vi "TAN to p2.vi"() -> ()   [LabVIEW 2009]
uses:
  <vilib>/printing/ReportDocExtensions.llb/Append Front Panel Image to Report (path).vi
  <vilib>/Utility/NIReport.llb/NI_report.lvclass
  <vilib>/Utility/NIReport.llb/NI_ReportGenerationCore.lvlib
panel:
  in  "Tab Control":enum32{"serving", "Receiving"}(tab)
  out "ALL":dbl[](graph)
  out "Left 2":dbl[](graph)
  out "Right 2":dbl[](graph)
  out "Serve 4":dbl[](graph)
  out "Serve 5":dbl[](graph)
  out "Serve 1":dbl[](graph)
  out "Serve 6":dbl[](graph)
  out "Serve 7":dbl[](graph)
  out "Serve 2":dbl[](graph)
  out "Serve 8":dbl[](graph)
  out "Serve 9":dbl[](graph)
  out "Serve 3":dbl[](graph)
  in  "S1":bool
  in  "TL":bool
  in  "BR":bool
  in  "BL":bool
  in  "BM":bool
  in  "CR":bool
  in  "CM":bool
  in  "CL":bool
  in  "TR":bool
  in  "TM":bool
  in  "1":bool
  in  "2":bool
  in  "3":bool
  in  "S 2":bool
  in  "Code":bool
  in  "stop":bool
  in  "save file to":path=path "C:/Users/Sports Tech/Desktop/kokum/Service VI/SAVED FILES/results.doc"
  in  "String":string
  in  "reset":bool
  in  "Boolean":bool
  in  "TM 3":bool
  in  "TR 3":bool
  in  "CL 3":bool
  in  "CM 3":bool
  in  "CR  3":bool
  in  "BM 3":bool
  in  "BL 3":bool
  in  "BR 3":bool
  in  "TL 3":bool
  in  "TM 2":bool
  in  "TR 2":bool
  in  "CL 2":bool
  in  "CM 2":bool
  in  "CR  2":bool
  in  "BM 2":bool
  in  "BL 2":bool
  in  "BR 2":bool
  in  "TL 2":bool
  out "All":dbl[](graph)
  out "Right":dbl[](graph)
  out "Left":dbl[](graph)
  out "Return 6":dbl[](graph)
  out "return to 9":dbl[](graph)
  out "return to 6":dbl[](graph)
  out "Return 7":dbl[](graph)
  out "return to 10":dbl[](graph)
  out "return to 7":dbl[](graph)
  out "Return 8":dbl[](graph)
  out "return to 11":dbl[](graph)
  out "return to 8":dbl[](graph)
  out "Return 0":dbl[](graph)
  out "return to 3":dbl[](graph)
  out "return to 0":dbl[](graph)
  out "Return 1":dbl[](graph)
  out "return to 4":dbl[](graph)
  out "return to 1":dbl[](graph)
  out "Return 2":dbl[](graph)
  out "return to 5":dbl[](graph)
  out "return to 2":dbl[](graph)
  out "return to 1 from right":dbl[][](array[numeric])
  out "return to 2 from right":dbl[][](array[numeric])
  out "return to 6 from right":dbl[][](array[numeric])
  out "return to 7 from right":dbl[][](array[numeric])
  out "return to 8 from right":dbl[][](array[numeric])
  out "return to 0 from right":dbl[][](array[numeric])
  out "return to 8 from left":dbl[][](array[numeric])
  out "return to 7 from left":dbl[][](array[numeric])
  out "return to 6 from left":dbl[][](array[numeric])
  out "return to 2 from left":dbl[][](array[numeric])
  out "return to 1 from left":dbl[][](array[numeric])
  out "return to 0 from left":dbl[][](array[numeric])
  out "All receives":dbl[][](array[numeric])
  out "receive from left":dbl[][](array[numeric])
  out "receive from right":dbl[][](array[numeric])
  out "serve3":dbl[][](array[numeric])
  out "serve2":dbl[][](array[numeric])
  out "serve1":dbl[][](array[numeric])
  out "serv1 from right":dbl[][](array[numeric])
  out "serv2 from right":dbl[][](array[numeric])
  out "serv3 from right":dbl[][](array[numeric])
  out "serv3 from left":dbl[][](array[numeric])
  out "serv2 from left":dbl[][](array[numeric])
  out "serv1 from left":dbl[][](array[numeric])
  out "all serves":dbl[][](array[numeric])
  out "service from right":dbl[][](array[numeric])
  out "serving from left":dbl[][](array[numeric])
  # "SWITCH"
  # "Receiving"
  # "Player position"
  # "Serving"
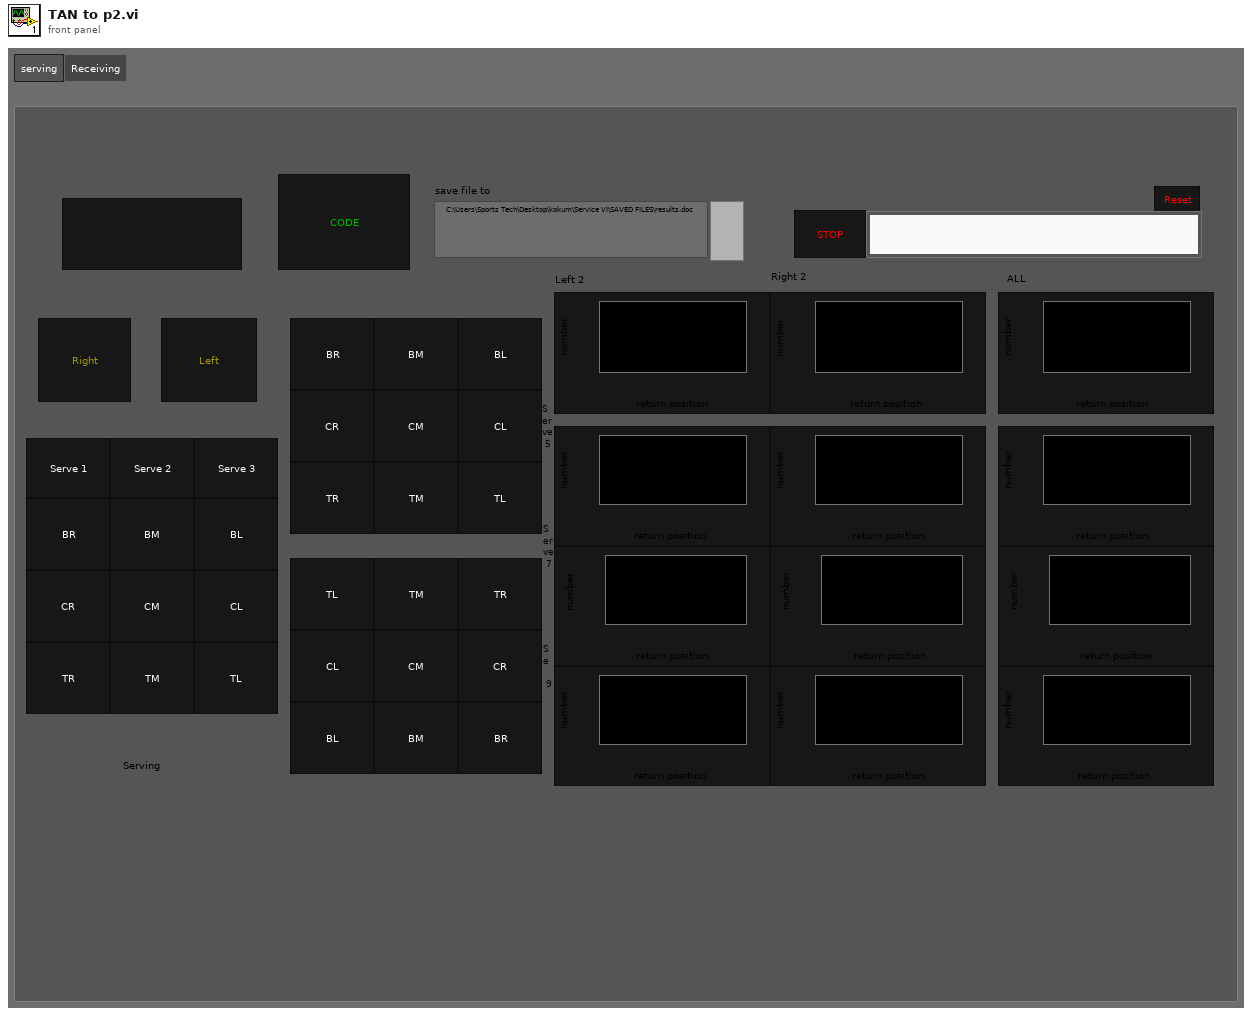
[diagram p1: front panel]
types:
  T1 = typedef "LVPositionTypeDef.ctl" = cluster{"Left":i32, "Top":i32}
  T2 = cluster{"Position":T1, "Position":T1, "Position":T1, "Position":T1, "Position":T1, "Position":T1, "Position":T1, "Position":T1, "Position":T1}
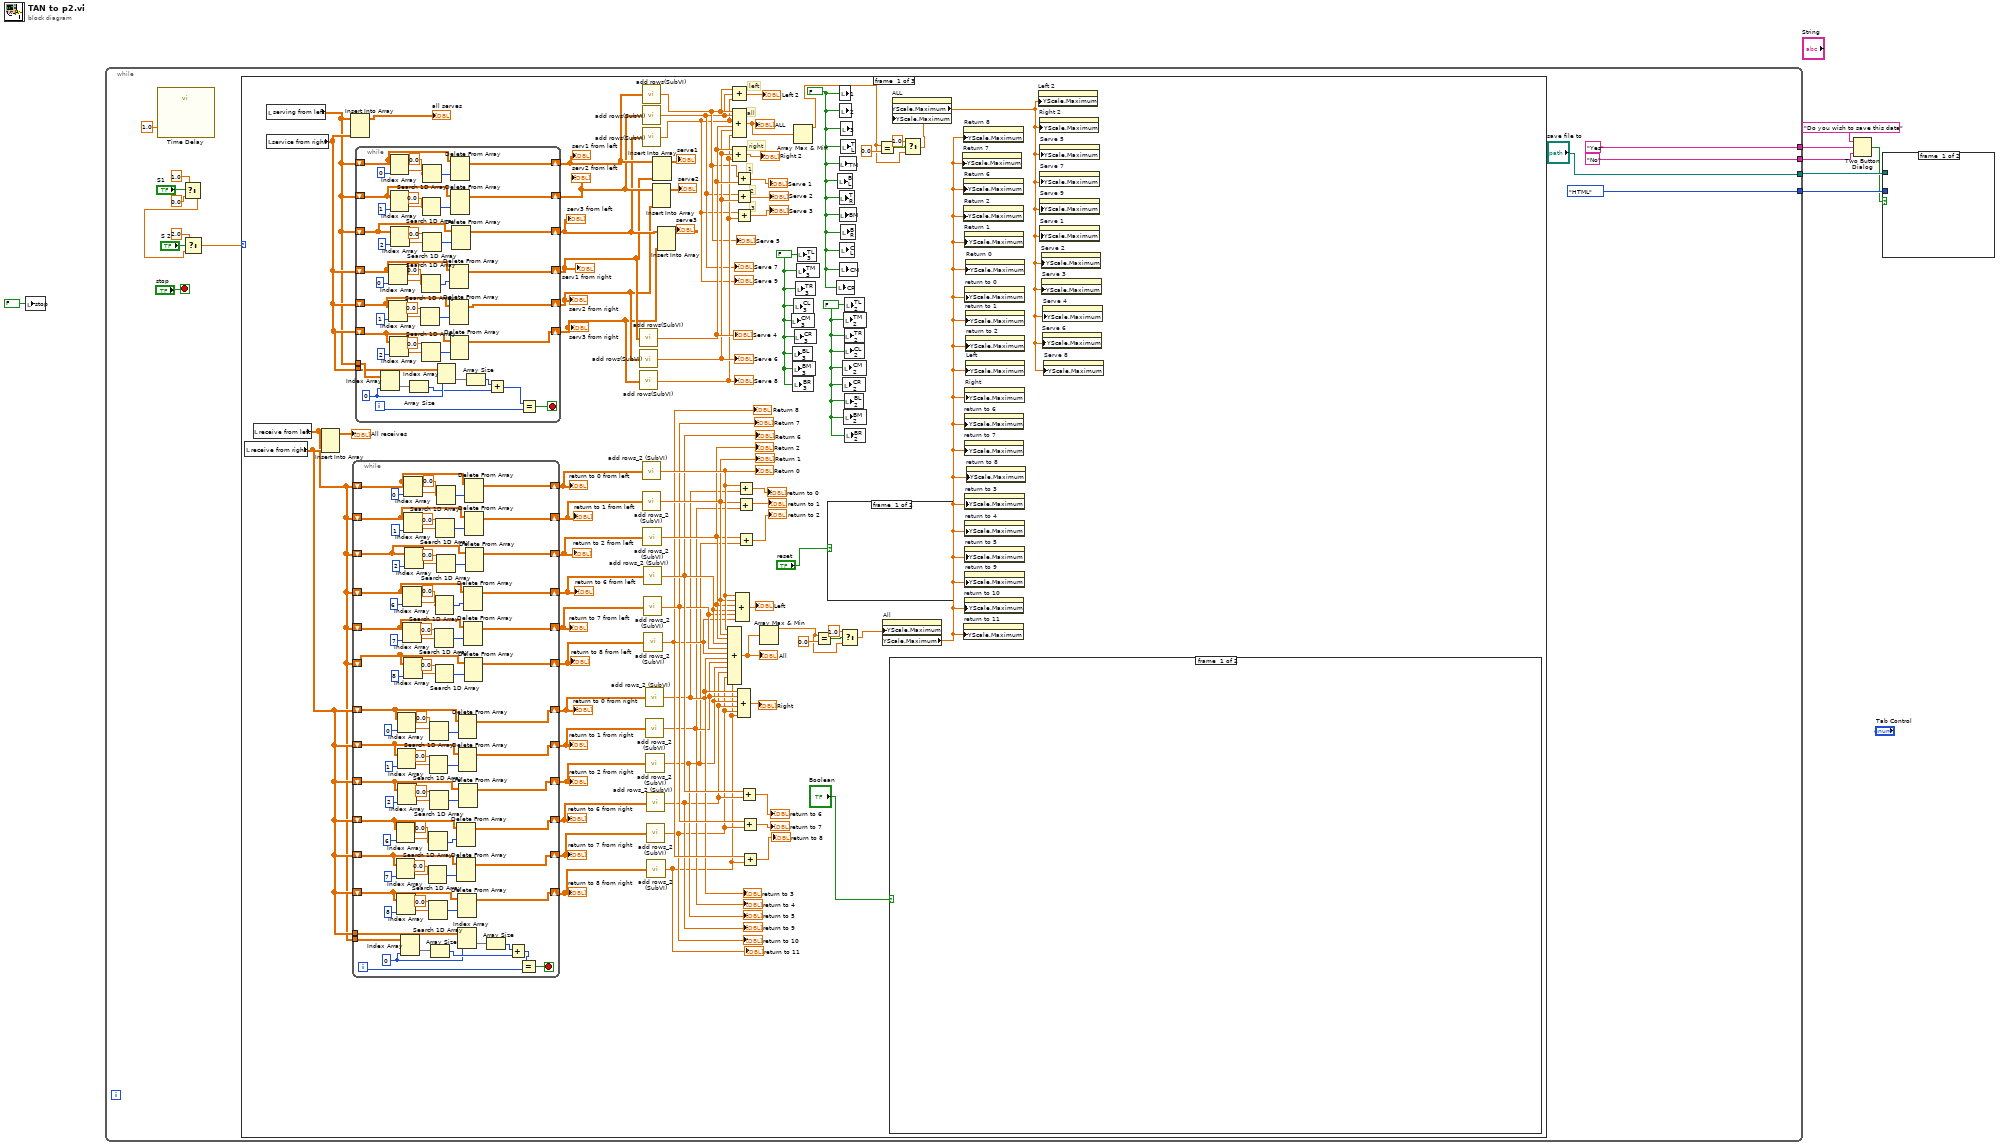
[diagram p0: block diagram]
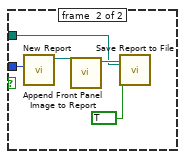
[diagram p2: hidden frame]
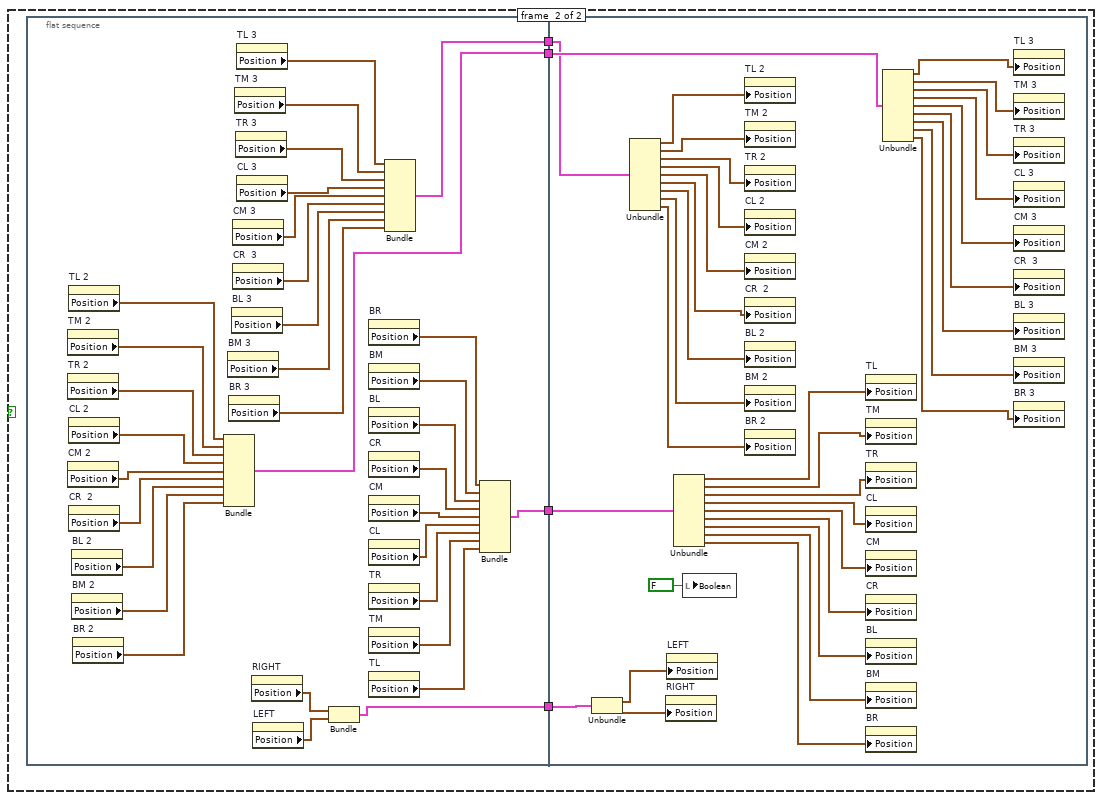
[diagram p3: hidden frame]
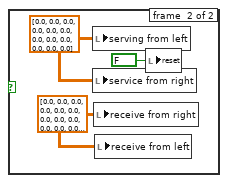
[diagram p4: hidden frame]
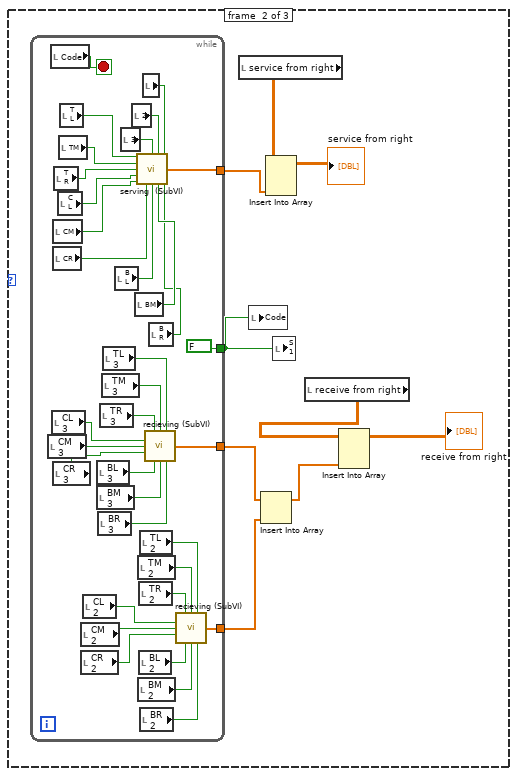
[diagram p5: hidden frame]
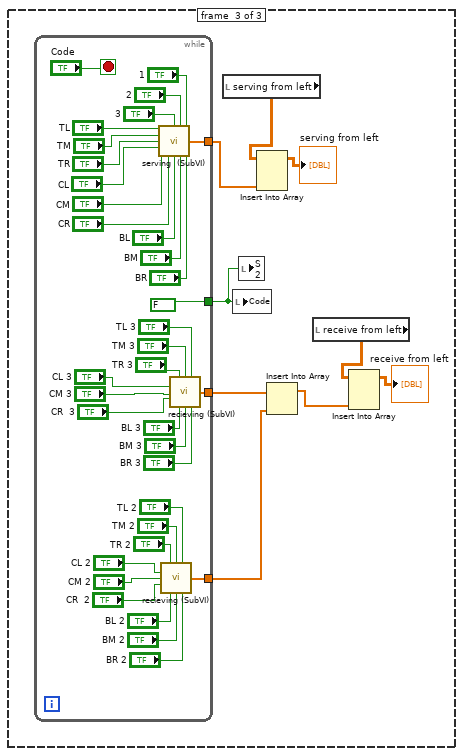
[diagram p6: hidden frame]
diagram:
  n1 = local write "stop"(FALSE ("stop")) -> ()
  n2 = while {
    tunnel: [enum16{"Standard Report", "HTML"}."HTML" ("report type")] -> w7
    tunnel: ["save file to"] -> w6
    tunnel: ["Yes" ("T button name (\"OK\")")] -> w3
    tunnel: ["No" ("F button name (\"Cancel\")")] -> w2
    stop <- "stop" stop-if-true
    n3 = call "Time Delay"("Delay Time (s)"=1.0) -> ()  [unwired: 10 in, 1 out]
    n4 = Select(t=1.0, s="S1", f=0.0) -> (s? t:f=w15:dbl)
    n5 = Select(t=2.0, s="S 2", f=w15) -> (s? t:f=w13:dbl)
    n6 = case shown="0, Default" w13 {
      frame #0 {
        w73 = FALSE ("TL 3")
        w72 = FALSE ("TL 3")
        w74 = FALSE ("1")
        # "3"
        # "2"
        # "1"
        # "all"
        # "right"
        # "left"
        n7 = local read "receive from right"() -> (w70:dbl[][])
        n8 = local read "receive from left"() -> (w69:dbl[][])
        n9 = local read "service from right"() -> (w97:dbl[][])
        n10 = local read "serving from left"() -> (w92:dbl[][])
        n11 = Insert Into Array(array=w69, new element=w70) -> (→"All receives":dbl[][])  [unwired: 2 in]
        n12 = Insert Into Array(array=w92, new element=w97) -> (→"all serves":dbl[][])  [unwired: 2 in]
        n13 = while {
          shift-right: [w223] -> w68
          shift-left: w69 -> [w229]
          shift-right: [w222] -> w67
          shift-left: w69 -> [w228]
          shift-right: [w221] -> w66
          shift-left: w69 -> [w227]
          shift-right: [w220] -> w65
          shift-left: w69 -> [w226]
          shift-right: [w219] -> w64
          shift-left: w69 -> [w225]
          shift-right: [w218] -> w63
          shift-left: w69 -> [w224]
          shift-right: [w187] -> w62
          shift-left: w70 -> [w193]
          shift-right: [w186] -> w61
          shift-left: w70 -> [w192]
          shift-right: [w185] -> w60
          shift-left: w70 -> [w188]
          shift-right: [w184] -> w59
          shift-left: w70 -> [w191]
          shift-right: [w183] -> w58
          shift-left: w70 -> [w190]
          shift-right: [w182] -> w57
          shift-left: w70 -> [w189]
          tunnel: w70 -> [w176]
          tunnel: w69 -> [w175]
          i -> [w173]
          stop <- w172 stop-if-true
          w177 = 0 ("disabled index (col)")
          n14 = Index Array(array=w191, index (col)=6 ("disabled index (col)")) -> (element=w194:dbl[])  [unwired: 1 in]
          n15 = Index Array(array=w190, index (col)=7 ("disabled index (col)")) -> (element=w199:dbl[])  [unwired: 1 in]
          n16 = Index Array(array=w189, index (col)=8 ("disabled index (col)")) -> (element=w205:dbl[])  [unwired: 1 in]
          n17 = Index Array(array=w193, index (col)=0 ("disabled index (col)")) -> (element=w217:dbl[])  [unwired: 1 in]
          n18 = Index Array(array=w192, index (col)=1 ("disabled index (col)")) -> (element=w212:dbl[])  [unwired: 1 in]
          n19 = Index Array(array=w188, index (col)=2 ("disabled index (col)")) -> (element=w206:dbl[])  [unwired: 1 in]
          n20 = Index Array(array=w175, index (col)=w177) -> (element=w180:dbl[])  [unwired: 1 in]
          n21 = Index Array(array=w226, index (col)=6 ("disabled index (col)")) -> (element=w253:dbl[])  [unwired: 1 in]
          n22 = Index Array(array=w225, index (col)=7 ("disabled index (col)")) -> (element=w248:dbl[])  [unwired: 1 in]
          n23 = Index Array(array=w224, index (col)=8 ("disabled index (col)")) -> (element=w242:dbl[])  [unwired: 1 in]
          n24 = Index Array(array=w229, index (col)=0 ("disabled index (col)")) -> (element=w230:dbl[])  [unwired: 1 in]
          n25 = Index Array(array=w228, index (col)=1 ("disabled index (col)")) -> (element=w235:dbl[])  [unwired: 1 in]
          n26 = Index Array(array=w227, index (col)=2 ("disabled index (col)")) -> (element=w241:dbl[])  [unwired: 1 in]
          n27 = Search 1D Array(1D array=w199, element=0.0) -> (index of element=w197:i32)  [unwired: 1 in]
          n28 = Search 1D Array(1D array=w194, element=0.0) -> (index of element=w196:i32)  [unwired: 1 in]
          n29 = Search 1D Array(1D array=w205, element=0.0) -> (index of element=w203:i32)  [unwired: 1 in]
          n30 = Search 1D Array(1D array=w212, element=0.0) -> (index of element=w214:i32)  [unwired: 1 in]
          n31 = Search 1D Array(1D array=w217, element=0.0) -> (index of element=w215:i32)  [unwired: 1 in]
          n32 = Search 1D Array(1D array=w206, element=0.0) -> (index of element=w208:i32)  [unwired: 1 in]
          n33 = Array Size(array=w180) -> (size(s)=w178:i32)
          n34 = Search 1D Array(1D array=w248, element=0.0) -> (index of element=w250:i32)  [unwired: 1 in]
          n35 = Search 1D Array(1D array=w253, element=0.0) -> (index of element=w251:i32)  [unwired: 1 in]
          n36 = Search 1D Array(1D array=w242, element=0.0) -> (index of element=w244:i32)  [unwired: 1 in]
          n37 = Search 1D Array(1D array=w235, element=0.0) -> (index of element=w233:i32)  [unwired: 1 in]
          n38 = Search 1D Array(1D array=w230, element=0.0) -> (index of element=w232:i32)  [unwired: 1 in]
          n39 = Search 1D Array(1D array=w241, element=0.0) -> (index of element=w239:i32)  [unwired: 1 in]
          n40 = Delete From Array(array=w191, index (row)=w196) -> (array with subset deleted=w184:dbl[][])  [unwired: 2 in, 1 out]
          n41 = Delete From Array(array=w190, index (row)=w197) -> (array with subset deleted=w183:dbl[][])  [unwired: 2 in, 1 out]
          n42 = Delete From Array(array=w189, index (row)=w203) -> (array with subset deleted=w182:dbl[][])  [unwired: 2 in, 1 out]
          n43 = Index Array(array=w176, index (col)=w177) -> (element=w181:dbl[])  [unwired: 1 in]
          n44 = Delete From Array(array=w193, index (row)=w215) -> (array with subset deleted=w187:dbl[][])  [unwired: 2 in, 1 out]
          n45 = Delete From Array(array=w192, index (row)=w214) -> (array with subset deleted=w186:dbl[][])  [unwired: 2 in, 1 out]
          n46 = Delete From Array(array=w188, index (row)=w208) -> (array with subset deleted=w185:dbl[][])  [unwired: 2 in, 1 out]
          n47 = Delete From Array(array=w226, index (row)=w251) -> (array with subset deleted=w220:dbl[][])  [unwired: 2 in, 1 out]
          n48 = Delete From Array(array=w225, index (row)=w250) -> (array with subset deleted=w219:dbl[][])  [unwired: 2 in, 1 out]
          n49 = Delete From Array(array=w224, index (row)=w244) -> (array with subset deleted=w218:dbl[][])  [unwired: 2 in, 1 out]
          n50 = Delete From Array(array=w229, index (row)=w232) -> (array with subset deleted=w223:dbl[][])  [unwired: 2 in, 1 out]
          n51 = Delete From Array(array=w228, index (row)=w233) -> (array with subset deleted=w222:dbl[][])  [unwired: 2 in, 1 out]
          n52 = Delete From Array(array=w227, index (row)=w239) -> (array with subset deleted=w221:dbl[][])  [unwired: 2 in, 1 out]
          n53 = Array Size(array=w181) -> (size(s)=w179:i32)
          n54 = Add(x=w179, y=w178) -> (x+y=w174:i32)
          n55 = Equal?(x=w174, y=w173) -> (x = y?=w172:bool)
        }
        "return to 0 from left" <- w68
        "return to 1 from left" <- w67
        "return to 2 from left" <- w66
        "return to 6 from left" <- w65
        "return to 7 from left" <- w64
        "return to 8 from left" <- w63
        "return to 0 from right" <- w62
        "return to 1 from right" <- w61
        "return to 2 from right" <- w60
        "return to 6 from right" <- w59
        "return to 7 from right" <- w58
        "return to 8 from right" <- w57
        n56 = while {
          shift-right: [w295] -> w91
          shift-left: w92 -> [w297]
          shift-right: [w288] -> w90
          shift-left: w92 -> [w289]
          shift-right: [w283] -> w89
          shift-left: w92 -> [w284]
          shift-right: [w263] -> w88
          shift-left: w97 -> [w266]
          shift-right: [w262] -> w87
          shift-left: w97 -> [w265]
          shift-right: [w261] -> w86
          shift-left: w97 -> [w264]
          tunnel: w92 -> [w260]
          tunnel: w97 -> [w258]
          i -> [w281]
          stop <- w280 stop-if-true
          w259 = 0 ("disabled index (col)")
          n57 = Index Array(array=w260, index (col)=w259) -> (element=w257:dbl[])  [unwired: 1 in]
          n58 = Index Array(array=w266, index (col)=0 ("disabled index (col)")) -> (element=w267:dbl[])  [unwired: 1 in]
          n59 = Index Array(array=w265, index (col)=1 ("disabled index (col)")) -> (element=w272:dbl[])  [unwired: 1 in]
          n60 = Index Array(array=w264, index (col)=2 ("disabled index (col)")) -> (element=w278:dbl[])  [unwired: 1 in]
          n61 = Index Array(array=w297, index (col)=0 ("disabled index (col)")) -> (element=w299:dbl[])  [unwired: 1 in]
          n62 = Index Array(array=w289, index (col)=1 ("disabled index (col)")) -> (element=w292:dbl[])  [unwired: 1 in]
          n63 = Index Array(array=w284, index (col)=2 ("disabled index (col)")) -> (element=w282:dbl[])  [unwired: 1 in]
          n64 = Array Size(array=w257) -> (size(s)=w255:i32)
          n65 = Search 1D Array(1D array=w272, element=0.0) -> (index of element=w270:i32)  [unwired: 1 in]
          n66 = Search 1D Array(1D array=w267, element=0.0) -> (index of element=w269:i32)  [unwired: 1 in]
          n67 = Search 1D Array(1D array=w278, element=0.0) -> (index of element=w276:i32)  [unwired: 1 in]
          n68 = Search 1D Array(1D array=w292, element=0.0) -> (index of element=w294:i32)  [unwired: 1 in]
          n69 = Search 1D Array(1D array=w299, element=0.0) -> (index of element=w296:i32)  [unwired: 1 in]
          n70 = Search 1D Array(1D array=w282, element=0.0) -> (index of element=w286:i32)  [unwired: 1 in]
          n71 = Index Array(array=w258, index (col)=w259) -> (element=w279:dbl[])  [unwired: 1 in]
          n72 = Delete From Array(array=w266, index (row)=w269) -> (array with subset deleted=w263:dbl[][])  [unwired: 2 in, 1 out]
          n73 = Delete From Array(array=w265, index (row)=w270) -> (array with subset deleted=w262:dbl[][])  [unwired: 2 in, 1 out]
          n74 = Delete From Array(array=w264, index (row)=w276) -> (array with subset deleted=w261:dbl[][])  [unwired: 2 in, 1 out]
          n75 = Delete From Array(array=w297, index (row)=w296) -> (array with subset deleted=w295:dbl[][])  [unwired: 2 in, 1 out]
          n76 = Delete From Array(array=w289, index (row)=w294) -> (array with subset deleted=w288:dbl[][])  [unwired: 2 in, 1 out]
          n77 = Delete From Array(array=w284, index (row)=w286) -> (array with subset deleted=w283:dbl[][])  [unwired: 2 in, 1 out]
          n78 = Array Size(array=w279) -> (size(s)=w256:i32)
          n79 = Add(x=w256, y=w255) -> (x+y=w254:i32)
          n80 = Equal?(x=w254, y=w281) -> (x = y?=w280:bool)
        }
        "serv1 from left" <- w91
        "serv2 from left" <- w90
        "serv3 from left" <- w89
        "serv1 from right" <- w88
        "serv2 from right" <- w87
        "serv3 from right" <- w86
        n81 = call "add rows(SubVI).vi"("array in"=w88) -> ("array out"=w85:dbl[])
        "Serve 4" <- w85
        n82 = call "add rows(SubVI).vi"("array in"=w87) -> ("array out"=w84:dbl[])
        "Serve 6" <- w84
        n83 = call "add rows(SubVI).vi"("array in"=w86) -> ("array out"=w83:dbl[])
        "Serve 8" <- w83
        n84 = call "add rows(SubVI).vi"("array in"=w91) -> ("array out"=w82:dbl[])
        "Serve 5" <- w82
        n85 = call "add rows(SubVI).vi"("array in"=w90) -> ("array out"=w81:dbl[])
        "Serve 7" <- w81
        n86 = call "add rows(SubVI).vi"("array in"=w89) -> ("array out"=w80:dbl[])
        "Serve 9" <- w80
        n87 = call "add rows_2 (SubVI).vi"("array in"=w68) -> ("array out"=w56:dbl[])
        "Return 0" <- w56
        n88 = call "add rows_2 (SubVI).vi"("array in"=w67) -> ("array out"=w55:dbl[])
        "Return 1" <- w55
        n89 = call "add rows_2 (SubVI).vi"("array in"=w66) -> ("array out"=w54:dbl[])
        "Return 2" <- w54
        n90 = call "add rows_2 (SubVI).vi"("array in"=w65) -> ("array out"=w53:dbl[])
        "Return 6" <- w53
        n91 = call "add rows_2 (SubVI).vi"("array in"=w64) -> ("array out"=w52:dbl[])
        "Return 7" <- w52
        n92 = call "add rows_2 (SubVI).vi"("array in"=w63) -> ("array out"=w51:dbl[])
        "Return 8" <- w51
        n93 = call "add rows_2 (SubVI).vi"("array in"=w62) -> ("array out"=w50:dbl[])
        "return to 3" <- w50
        n94 = call "add rows_2 (SubVI).vi"("array in"=w61) -> ("array out"=w49:dbl[])
        "return to 4" <- w49
        n95 = call "add rows_2 (SubVI).vi"("array in"=w60) -> ("array out"=w48:dbl[])
        "return to 5" <- w48
        n96 = call "add rows_2 (SubVI).vi"("array in"=w59) -> ("array out"=w47:dbl[])
        "return to 9" <- w47
        n97 = call "add rows_2 (SubVI).vi"("array in"=w58) -> ("array out"=w46:dbl[])
        "return to 10" <- w46
        n98 = call "add rows_2 (SubVI).vi"("array in"=w57) -> ("array out"=w45:dbl[])
        "return to 11" <- w45
        n99 = Insert Into Array(array=w90, new element=w87) -> (→"serve2":dbl[][])  [unwired: 2 in]
        n100 = Insert Into Array(array=w91, new element=w88) -> (→"serve1":dbl[][])  [unwired: 2 in]
        n101 = Insert Into Array(array=w89, new element=w86) -> (→"serve3":dbl[][])  [unwired: 2 in]
        n102 = Compound Arithmetic op=ADD(w56, w55, w54, w53, w52, w51, w50, w49, w48, w47, w46, w45) -> (w35:dbl[])
        "All" <- w35
        n103 = Compound Arithmetic op=ADD(w82, w81, w80, w85, w84, w83) -> (w33:dbl[])
        "ALL" <- w33
        n104 = Compound Arithmetic op=ADD(w85, w84, w83) -> (→"Right 2":dbl[])
        n105 = Compound Arithmetic op=ADD(w82, w81, w80) -> (→"Left 2":dbl[])
        n106 = Add(x=w82, y=w85) -> (x+y=→"Serve 1":dbl[])
        n107 = Add(x=w81, y=w84) -> (x+y=→"Serve 2":dbl[])
        n108 = Add(x=w80, y=w83) -> (x+y=→"Serve 3":dbl[])
        n109 = Compound Arithmetic op=ADD(w56, w55, w54, w53, w52, w51) -> (→"Left":dbl[])
        n110 = Add(x=w56, y=w50) -> (x+y=→"return to 0":dbl[])
        n111 = Add(x=w55, y=w49) -> (x+y=→"return to 1":dbl[])
        n112 = Add(x=w54, y=w48) -> (x+y=→"return to 2":dbl[])
        n113 = Compound Arithmetic op=ADD(w50, w49, w48, w47, w46, w45) -> (→"Right":dbl[])
        n114 = Add(x=w53, y=w47) -> (x+y=→"return to 6":dbl[])
        n115 = Add(x=w52, y=w46) -> (x+y=→"return to 7":dbl[])
        n116 = Add(x=w51, y=w45) -> (x+y=→"return to 8":dbl[])
        n117 = Array Max & Min(array=w35) -> (max value=w24:dbl)  [unwired: 3 out]
        n118 = local write "CM 3"(w72) -> ()
        n119 = local write "BL 3"(w72) -> ()
        n120 = local write "BM 3"(w72) -> ()
        n121 = local write "BR 3"(w72) -> ()
        n122 = Array Max & Min(array=w33) -> (max value=w29:dbl)  [unwired: 3 out]
        n123 = local write "CL 3"(w72) -> ()
        n124 = local write "CR  3"(w72) -> ()
        n125 = local write "TR 3"(w72) -> ()
        n126 = local write "TM 3"(w72) -> ()
        n127 = local write "TL 3"(w72) -> ()
        n128 = Equal?(x=w24, y=0.0) -> (x = y?=w26:bool)
        n129 = case shown="True" "reset" {
          frame #0 {
          }
          frame #1 {
            w171 = dbl[][] [[0.0, 0.0, 0.0, 0.0, 0.0, 0.0, 0.0, 0.0, 0.0, 0.0, 0.0, 0.0, 0.0, 0.0, 0.0, 0.0, 0.0, 0.0]] ("serving from left")
            w170 = dbl[][] [[0.0, 0.0, 0.0, 0.0, 0.0, 0.0, 0.0, 0.0, 0.0, 0.0, 0.0, 0.0]] ("serving from left")
            n130 = local write "serving from left"(w170) -> ()
            n131 = local write "service from right"(w170) -> ()
            n132 = local write "receive from right"(w171) -> ()
            n133 = local write "receive from left"(w171) -> ()
            n134 = local write "reset"(FALSE ("reset")) -> ()
          }
        }
        n135 = local write "CR"(w74) -> ()
        n136 = local write "BL"(w74) -> ()
        n137 = local write "TM"(w74) -> ()
        n138 = local write "TR"(w74) -> ()
        n139 = local write "BM"(w74) -> ()
        n140 = local write "1"(w74) -> ()
        n141 = local write "2"(w74) -> ()
        n142 = local write "CL"(w74) -> ()
        n143 = local write "CM"(w74) -> ()
        n144 = local write "3"(w74) -> ()
        n145 = local write "BR"(w74) -> ()
        n146 = Select(t=1.0, s=w26, f=w24) -> (s? t:f=w23:dbl)
        n147 = local write "TL"(w74) -> ()
        n148 = local write "CM 2"(w73) -> ()
        n149 = local write "CR  2"(w73) -> ()
        n150 = local write "TM 2"(w73) -> ()
        n151 = local write "BM 2"(w73) -> ()
        n152 = local write "TR 2"(w73) -> ()
        n153 = local write "CL 2"(w73) -> ()
        n154 = local write "BL 2"(w73) -> ()
        n155 = local write "TL 2"(w73) -> ()
        n156 = local write "BR 2"(w73) -> ()
        n157 = Equal?(x=w29, y=0.0) -> (x = y?=w31:bool)
        n158 = property on="All" class="WFGraph (strict)"("YScale.Maximum"=w23) -> ("YScale.Maximum"=w34:dbl)  [unwired: 2 in, 2 out]
        n159 = case shown="True" "Boolean" {
          frame #0 {
          }
          frame #1 {
            n160 = flat-sequence {
              tunnel: [w105] -> w101
              tunnel: [w104] -> w100
              tunnel: [w103] -> w99
              tunnel: [w102] -> w98
              tunnel: w101 -> [w158]
              tunnel: w100 -> [w168]
              tunnel: w99 -> [w148]
              tunnel: w98 -> [w138]
              frame #0 {
                n161 = property on="TM 2" class="Bool (strict)"() -> ("Position"=w124:T1)  [unwired: 2 in, 2 out]
                n162 = property on="TR 2" class="Bool (strict)"() -> ("Position"=w123:T1)  [unwired: 2 in, 2 out]
                n163 = property on="CM 2" class="Bool (strict)"() -> ("Position"=w121:T1)  [unwired: 2 in, 2 out]
                n164 = property on="TL 2" class="Bool (strict)"() -> ("Position"=w125:T1)  [unwired: 2 in, 2 out]
                n165 = property on="CL 2" class="Bool (strict)"() -> ("Position"=w122:T1)  [unwired: 2 in, 2 out]
                n166 = property on="CR  2" class="Bool (strict)"() -> ("Position"=w120:T1)  [unwired: 2 in, 2 out]
                n167 = property on="BL 2" class="Bool (strict)"() -> ("Position"=w119:T1)  [unwired: 2 in, 2 out]
                n168 = property on="BM 2" class="Bool (strict)"() -> ("Position"=w118:T1)  [unwired: 2 in, 2 out]
                n169 = property on="BR 2" class="Bool (strict)"() -> ("Position"=w117:T1)  [unwired: 2 in, 2 out]
                n170 = Bundle("Position"=w125, "Position"=w124, "Position"=w123, "Position"=w122, "Position"=w121, "Position"=w120, "Position"=w119, "Position"=w118, "Position"=w117) -> (w104:T2)  [unwired: 1 in]
                n171 = property on="BM 3" class="Bool (strict)"() -> ("Position"=w127:T1)  [unwired: 2 in, 2 out]
                n172 = property on="BR 3" class="Bool (strict)"() -> ("Position"=w126:T1)  [unwired: 2 in, 2 out]
                n173 = property on="BL 3" class="Bool (strict)"() -> ("Position"=w128:T1)  [unwired: 2 in, 2 out]
                n174 = property on="CM 3" class="Bool (strict)"() -> ("Position"=w130:T1)  [unwired: 2 in, 2 out]
                n175 = property on="CR  3" class="Bool (strict)"() -> ("Position"=w129:T1)  [unwired: 2 in, 2 out]
                n176 = property on="TM 3" class="Bool (strict)"() -> ("Position"=w133:T1)  [unwired: 2 in, 2 out]
                n177 = property on="TR 3" class="Bool (strict)"() -> ("Position"=w132:T1)  [unwired: 2 in, 2 out]
                n178 = property on="TL 3" class="Bool (strict)"() -> ("Position"=w134:T1)  [unwired: 2 in, 2 out]
                n179 = property on="CL 3" class="Bool (strict)"() -> ("Position"=w131:T1)  [unwired: 2 in, 2 out]
                n180 = property on="RIGHT" class="Bool (strict)"() -> ("Position"=w106:T1)  [unwired: 2 in, 2 out]
                n181 = property on="LEFT" class="Bool (strict)"() -> ("Position"=w107:T1)  [unwired: 2 in, 2 out]
                n182 = Bundle("Position"=w106, "Position"=w107) -> (w102:cluster{"Position":T1, "Position":T1})  [unwired: 1 in]
                n183 = property on="BR" class="Bool (strict)"() -> ("Position"=w116:T1)  [unwired: 2 in, 2 out]
                n184 = property on="BM" class="Bool (strict)"() -> ("Position"=w115:T1)  [unwired: 2 in, 2 out]
                n185 = property on="BL" class="Bool (strict)"() -> ("Position"=w114:T1)  [unwired: 2 in, 2 out]
                n186 = property on="CR" class="Bool (strict)"() -> ("Position"=w113:T1)  [unwired: 2 in, 2 out]
                n187 = property on="CM" class="Bool (strict)"() -> ("Position"=w112:T1)  [unwired: 2 in, 2 out]
                n188 = property on="CL" class="Bool (strict)"() -> ("Position"=w111:T1)  [unwired: 2 in, 2 out]
                n189 = property on="TR" class="Bool (strict)"() -> ("Position"=w110:T1)  [unwired: 2 in, 2 out]
                n190 = property on="TM" class="Bool (strict)"() -> ("Position"=w109:T1)  [unwired: 2 in, 2 out]
                n191 = property on="TL" class="Bool (strict)"() -> ("Position"=w108:T1)  [unwired: 2 in, 2 out]
                n192 = Bundle("Position"=w134, "Position"=w133, "Position"=w132, "Position"=w131, "Position"=w130, "Position"=w129, "Position"=w128, "Position"=w127, "Position"=w126) -> (w105:T2)  [unwired: 1 in]
                n193 = Bundle("Position"=w116, "Position"=w115, "Position"=w114, "Position"=w113, "Position"=w112, "Position"=w111, "Position"=w110, "Position"=w109, "Position"=w108) -> (w103:T2)  [unwired: 1 in]
              }
              frame #1 {
                n194 = Unbundle(w138) -> ("Position"=w137:T1, "Position"=w136:T1)
                n195 = Unbundle(w158) -> ("Position"=w157:T1, "Position"=w156:T1, "Position"=w155:T1, "Position"=w154:T1, "Position"=w153:T1, "Position"=w152:T1, "Position"=w151:T1, "Position"=w150:T1, "Position"=w149:T1)
                n196 = property on="RIGHT" class="Bool (strict)"("Position"=w136) -> ()  [unwired: 2 in, 2 out]
                n197 = property on="LEFT" class="Bool (strict)"("Position"=w137) -> ()  [unwired: 2 in, 2 out]
                n198 = Unbundle(w148) -> ("Position"=w147:T1, "Position"=w146:T1, "Position"=w145:T1, "Position"=w144:T1, "Position"=w143:T1, "Position"=w142:T1, "Position"=w141:T1, "Position"=w140:T1, "Position"=w139:T1)
                n199 = local write "Boolean"(FALSE ("Boolean")) -> ()
                n200 = property on="TL 2" class="Bool (strict)"("Position"=w157) -> ()  [unwired: 2 in, 2 out]
                n201 = property on="TM 2" class="Bool (strict)"("Position"=w156) -> ()  [unwired: 2 in, 2 out]
                n202 = property on="TR 2" class="Bool (strict)"("Position"=w155) -> ()  [unwired: 2 in, 2 out]
                n203 = property on="CL 2" class="Bool (strict)"("Position"=w154) -> ()  [unwired: 2 in, 2 out]
                n204 = property on="CM 2" class="Bool (strict)"("Position"=w153) -> ()  [unwired: 2 in, 2 out]
                n205 = property on="CR  2" class="Bool (strict)"("Position"=w152) -> ()  [unwired: 2 in, 2 out]
                n206 = property on="BL 2" class="Bool (strict)"("Position"=w151) -> ()  [unwired: 2 in, 2 out]
                n207 = property on="BM 2" class="Bool (strict)"("Position"=w150) -> ()  [unwired: 2 in, 2 out]
                n208 = property on="BR 2" class="Bool (strict)"("Position"=w149) -> ()  [unwired: 2 in, 2 out]
                n209 = property on="TL" class="Bool (strict)"("Position"=w147) -> ()  [unwired: 2 in, 2 out]
                n210 = property on="TM" class="Bool (strict)"("Position"=w146) -> ()  [unwired: 2 in, 2 out]
                n211 = property on="TR" class="Bool (strict)"("Position"=w145) -> ()  [unwired: 2 in, 2 out]
                n212 = property on="CL" class="Bool (strict)"("Position"=w144) -> ()  [unwired: 2 in, 2 out]
                n213 = property on="CM" class="Bool (strict)"("Position"=w143) -> ()  [unwired: 2 in, 2 out]
                n214 = property on="CR" class="Bool (strict)"("Position"=w142) -> ()  [unwired: 2 in, 2 out]
                n215 = property on="BL" class="Bool (strict)"("Position"=w141) -> ()  [unwired: 2 in, 2 out]
                n216 = property on="BM" class="Bool (strict)"("Position"=w140) -> ()  [unwired: 2 in, 2 out]
                n217 = property on="BR" class="Bool (strict)"("Position"=w139) -> ()  [unwired: 2 in, 2 out]
                n218 = Unbundle(w168) -> ("Position"=w167:T1, "Position"=w166:T1, "Position"=w165:T1, "Position"=w164:T1, "Position"=w163:T1, "Position"=w162:T1, "Position"=w161:T1, "Position"=w160:T1, "Position"=w159:T1)
                n219 = property on="TL 3" class="Bool (strict)"("Position"=w167) -> ()  [unwired: 2 in, 2 out]
                n220 = property on="TM 3" class="Bool (strict)"("Position"=w166) -> ()  [unwired: 2 in, 2 out]
                n221 = property on="TR 3" class="Bool (strict)"("Position"=w165) -> ()  [unwired: 2 in, 2 out]
                n222 = property on="CL 3" class="Bool (strict)"("Position"=w164) -> ()  [unwired: 2 in, 2 out]
                n223 = property on="CM 3" class="Bool (strict)"("Position"=w163) -> ()  [unwired: 2 in, 2 out]
                n224 = property on="CR  3" class="Bool (strict)"("Position"=w162) -> ()  [unwired: 2 in, 2 out]
                n225 = property on="BL 3" class="Bool (strict)"("Position"=w161) -> ()  [unwired: 2 in, 2 out]
                n226 = property on="BM 3" class="Bool (strict)"("Position"=w160) -> ()  [unwired: 2 in, 2 out]
                n227 = property on="BR 3" class="Bool (strict)"("Position"=w159) -> ()  [unwired: 2 in, 2 out]
              }
            }
          }
        }
        n228 = Select(t=1.0, s=w31, f=w29) -> (s? t:f=w28:dbl)
        n229 = property on="ALL" class="WFGraph (strict)"("YScale.Maximum"=w28) -> ("YScale.Maximum"=w36:dbl)  [unwired: 2 in, 2 out]
        n230 = property on="Return 7" class="WFGraph (strict)"("YScale.Maximum"=w34) -> ()  [unwired: 2 in, 2 out]
        n231 = property on="Return 8" class="WFGraph (strict)"("YScale.Maximum"=w34) -> ()  [unwired: 2 in, 2 out]
        n232 = property on="Return 6" class="WFGraph (strict)"("YScale.Maximum"=w34) -> ()  [unwired: 2 in, 2 out]
        n233 = property on="Return 2" class="WFGraph (strict)"("YScale.Maximum"=w34) -> ()  [unwired: 2 in, 2 out]
        n234 = property on="return to 11" class="WFGraph (strict)"("YScale.Maximum"=w34) -> ()  [unwired: 2 in, 2 out]
        n235 = property on="Return 1" class="WFGraph (strict)"("YScale.Maximum"=w34) -> ()  [unwired: 2 in, 2 out]
        n236 = property on="return to 6" class="WFGraph (strict)"("YScale.Maximum"=w34) -> ()  [unwired: 2 in, 2 out]
        n237 = property on="return to 7" class="WFGraph (strict)"("YScale.Maximum"=w34) -> ()  [unwired: 2 in, 2 out]
        n238 = property on="return to 10" class="WFGraph (strict)"("YScale.Maximum"=w34) -> ()  [unwired: 2 in, 2 out]
        n239 = property on="return to 0" class="WFGraph (strict)"("YScale.Maximum"=w34) -> ()  [unwired: 2 in, 2 out]
        n240 = property on="Right" class="WFGraph (strict)"("YScale.Maximum"=w34) -> ()  [unwired: 2 in, 2 out]
        n241 = property on="return to 3" class="WFGraph (strict)"("YScale.Maximum"=w34) -> ()  [unwired: 2 in, 2 out]
        n242 = property on="return to 4" class="WFGraph (strict)"("YScale.Maximum"=w34) -> ()  [unwired: 2 in, 2 out]
        n243 = property on="return to 5" class="WFGraph (strict)"("YScale.Maximum"=w34) -> ()  [unwired: 2 in, 2 out]
        n244 = property on="return to 9" class="WFGraph (strict)"("YScale.Maximum"=w34) -> ()  [unwired: 2 in, 2 out]
        n245 = property on="Return 0" class="WFGraph (strict)"("YScale.Maximum"=w34) -> ()  [unwired: 2 in, 2 out]
        n246 = property on="return to 1" class="WFGraph (strict)"("YScale.Maximum"=w34) -> ()  [unwired: 2 in, 2 out]
        n247 = property on="return to 2" class="WFGraph (strict)"("YScale.Maximum"=w34) -> ()  [unwired: 2 in, 2 out]
        n248 = property on="Left" class="WFGraph (strict)"("YScale.Maximum"=w34) -> ()  [unwired: 2 in, 2 out]
        n249 = property on="return to 8" class="WFGraph (strict)"("YScale.Maximum"=w34) -> ()  [unwired: 2 in, 2 out]
        n250 = property on="Left 2" class="WFGraph (strict)"("YScale.Maximum"=w36) -> ()  [unwired: 2 in, 2 out]
        n251 = property on="Right 2" class="WFGraph (strict)"("YScale.Maximum"=w36) -> ()  [unwired: 2 in, 2 out]
        n252 = property on="Serve 5" class="WFGraph (strict)"("YScale.Maximum"=w36) -> ()  [unwired: 2 in, 2 out]
        n253 = property on="Serve 7" class="WFGraph (strict)"("YScale.Maximum"=w36) -> ()  [unwired: 2 in, 2 out]
        n254 = property on="Serve 9" class="WFGraph (strict)"("YScale.Maximum"=w36) -> ()  [unwired: 2 in, 2 out]
        n255 = property on="Serve 1" class="WFGraph (strict)"("YScale.Maximum"=w36) -> ()  [unwired: 2 in, 2 out]
        n256 = property on="Serve 2" class="WFGraph (strict)"("YScale.Maximum"=w36) -> ()  [unwired: 2 in, 2 out]
        n257 = property on="Serve 3" class="WFGraph (strict)"("YScale.Maximum"=w36) -> ()  [unwired: 2 in, 2 out]
        n258 = property on="Serve 6" class="WFGraph (strict)"("YScale.Maximum"=w36) -> ()  [unwired: 2 in, 2 out]
        n259 = property on="Serve 4" class="WFGraph (strict)"("YScale.Maximum"=w36) -> ()  [unwired: 2 in, 2 out]
        n260 = property on="Serve 8" class="WFGraph (strict)"("YScale.Maximum"=w36) -> ()  [unwired: 2 in, 2 out]
      }
      frame #1 {
        n261 = while {
          tunnel: [w331] -> w305
          tunnel: [FALSE ("S1")] -> w306
          tunnel: [w310] -> w302
          tunnel: [w309] -> w301
          stop <- w343 stop-if-true
          n262 = local read "CM 3"() -> (w324:bool)
          n263 = local read "Code"() -> (w343:bool)
          n264 = local read "CL 3"() -> (w323:bool)
          n265 = local read "CM"() -> (w338:bool)
          n266 = local read "CR"() -> (w339:bool)
          n267 = local read "CR  3"() -> (w325:bool)
          n268 = local read "TR"() -> (w329:bool)
          n269 = local read "CL"() -> (w337:bool)
          n270 = local read "TM"() -> (w336:bool)
          n271 = local read "TL"() -> (w335:bool)
          n272 = local read "CM 2"() -> (w315:bool)
          n273 = local read "CR  2"() -> (w316:bool)
          n274 = local read "CL 2"() -> (w314:bool)
          n275 = local read "BL 3"() -> (w326:bool)
          n276 = local read "BM 3"() -> (w327:bool)
          n277 = local read "BR 3"() -> (w328:bool)
          n278 = local read "TR 3"() -> (w322:bool)
          n279 = local read "TM 3"() -> (w321:bool)
          n280 = local read "TL 3"() -> (w320:bool)
          n281 = local read "BL"() -> (w342:bool)
          n282 = local read "3"() -> (w334:bool)
          n283 = local read "2"() -> (w333:bool)
          n284 = local read "BM"() -> (w341:bool)
          n285 = local read "TM 2"() -> (w312:bool)
          n286 = local read "BM 2"() -> (w318:bool)
          n287 = local read "TR 2"() -> (w313:bool)
          n288 = local read "BL 2"() -> (w317:bool)
          n289 = local read "TL 2"() -> (w311:bool)
          n290 = local read "BR 2"() -> (w319:bool)
          n291 = local read "1"() -> (w332:bool)
          n292 = call "recieving (SubVI).vi"("TR"=w322, "TM"=w321, "TL"=w320, "CL"=w323, "CM"=w324, "CR"=w325, "BL"=w326, "BM"=w327, "BR"=w328) -> ("appended array"=w310:dbl[])  [unwired: 6 in]
          n293 = local read "BR"() -> (w340:bool)
          n294 = call "serving  (SubVI).vi"("1"=w332, "BR"=w340, "2"=w333, "BM"=w341, "3"=w334, "BL"=w342, "CR"=w339, "TL"=w335, "TM"=w336, "TR"=w329, "CL"=w337, "CM"=w338) -> ("appended array"=w331:dbl[])  [unwired: 3 in]
          n295 = call "recieving (SubVI).vi"("TR"=w313, "TM"=w312, "TL"=w311, "CL"=w314, "CM"=w315, "CR"=w316, "BL"=w317, "BM"=w318, "BR"=w319) -> ("appended array"=w309:dbl[])  [unwired: 6 in]
        }
        n296 = local read "service from right"() -> (w307:dbl[][])
        n297 = local write "Code"(w306) -> ()
        n298 = Insert Into Array(array=w302, new element=w301) -> (w300:dbl[])  [unwired: 1 in]
        n299 = Insert Into Array(array=w307, new element=w305) -> (→"service from right":dbl[][])  [unwired: 2 in]
        n300 = local write "S1"(w306) -> ()
        n301 = local read "receive from right"() -> (w303:dbl[][])
        n302 = Insert Into Array(array=w303, new element=w300) -> (→"receive from right":dbl[][])  [unwired: 2 in]
      }
      frame #2 {
        n303 = while {
          tunnel: [w374] -> w350
          tunnel: [FALSE ("S 2")] -> w349
          tunnel: [w363] -> w346
          tunnel: [w353] -> w345
          stop <- "Code" stop-if-true
          n304 = call "serving  (SubVI).vi"("1"="1", "BR"="BR", "2"="2", "BM"="BM", "3"="3", "BL"="BL", "CR"="CR", "TL"="TL", "TM"="TM", "TR"="TR", "CL"="CL", "CM"="CM") -> ("appended array"=w374:dbl[])  [unwired: 3 in]
          n305 = call "recieving (SubVI).vi"("TR"="TR 2", "TM"="TM 2", "TL"="TL 2", "CL"="CL 2", "CM"="CM 2", "CR"="CR  2", "BL"="BL 2", "BM"="BM 2", "BR"="BR 2") -> ("appended array"=w353:dbl[])  [unwired: 6 in]
          n306 = call "recieving (SubVI).vi"("TR"="TR 3", "TM"="TM 3", "TL"="TL 3", "CL"="CL 3", "CM"="CM 3", "CR"="CR  3", "BL"="BL 3", "BM"="BM 3", "BR"="BR 3") -> ("appended array"=w363:dbl[])  [unwired: 6 in]
        }
        n307 = local read "serving from left"() -> (w351:dbl[][])
        n308 = local write "Code"(w349) -> ()
        n309 = local write "S 2"(w349) -> ()
        n310 = Insert Into Array(array=w351, new element=w350) -> (→"serving from left":dbl[][])  [unwired: 2 in]
        n311 = Insert Into Array(array=w346, new element=w345) -> (w344:dbl[])  [unwired: 1 in]
        n312 = local read "receive from left"() -> (w348:dbl[][])
        n313 = Insert Into Array(array=w348, new element=w344) -> (→"receive from left":dbl[][])  [unwired: 2 in]
      }
    }
  }
  n314 = Two Button Dialog(message="Do you wish to save this data", 1:w2, 2:w3) -> (T button?=w4:bool)
  n315 = case shown="True" w4 {
    tunnel: w7 -> [_ w392]
    tunnel: w6 -> [_ w389]
    frame #0 {
    }
    frame #1 {
      n316 = call <vilib>:"New Report.vi"("report type"=w392) -> ("report out"=w391:refnum<class "NI_report.lvclass">)  [unwired: 13 in, 1 out]
      n317 = call-poly <vilib>:"Append Front Panel Image to Report.vi"("report in"=w391) -> ("report out"=w390:refnum<class "NI_report.lvclass">)  [unwired: 10 in, 4 out]
      n318 = call-dynamic "Save Report to File.vi"("report in"=w390, "report file path"=w389, "prompt to replace? (F)"=TRUE ("Prompt to Replace? (F)")) -> ()  [unwired: 11 in, 2 out]
    }
  }
